vi "intiger to boolean Data.vi"(0 "data":u16[](array[numeric])) -> (3 "M":bool[](array[boolean]), 4 "M--- 0-7":bool[](array[boolean]), 6 "M--- 8-15":bool[](array[boolean]), 8 "M---16-23":bool[](array[boolean]), 10 "M--- 24-31":bool[](array[boolean]), 15 "M--- 32-39":bool[](array[boolean]))   [LabVIEW 2023]
panel:
  in  "?":u8
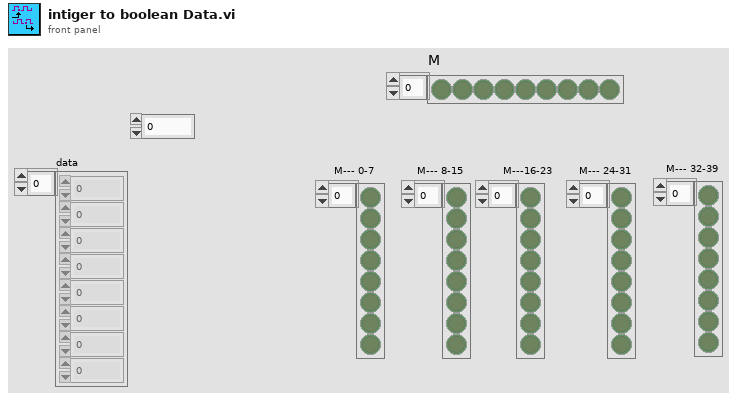
[diagram p1: front panel]
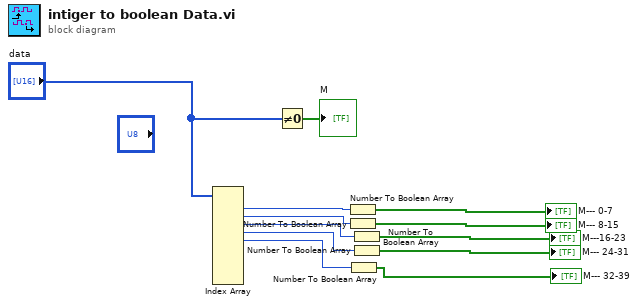
[diagram p0: block diagram]
diagram:
  n1 = Index Array(array="data") -> (element #1=w12:u16, element #2=w11:u16, element #3=w10:u16, element #4=w9:u16, element #5=w4:u16)  [unwired: 10 in, 5 out]
  n2 = Not Equal To 0?(x="data") -> (x != 0?=→"M":bool[])
  n3 = Number To Boolean Array(number=w12) -> (Boolean array=→"M--- 0-7":bool[])
  n4 = Number To Boolean Array(number=w11) -> (Boolean array=→"M--- 8-15":bool[])
  n5 = Number To Boolean Array(number=w4) -> (Boolean array=→"M--- 32-39":bool[])
  n6 = Number To Boolean Array(number=w10) -> (Boolean array=→"M---16-23":bool[])
  n7 = Number To Boolean Array(number=w9) -> (Boolean array=→"M--- 24-31":bool[])
